vi "Set Y Voltage.vi"(8 "error in (no error)":errorcluster, 10 "Set y Voltage(V)":dbl, 11 "hdl in":i32) -> (0 "error out":errorcluster, 3 "hdl":i32)   [LabVIEW 2011, in "Thorlabs_MDT69xB.lvlib"]
doc: "Set the output voltage for the Y axis."
uses:
  <instrlib>/Thorlabs_MDT69xB/Thorlabs_MDT69xB.lvlib
  <instrlib>/Thorlabs_MDT69xB/Data/MDT_COMMAND_LIB_win32.dll
  <instrlib>/Thorlabs_MDT69xB/Data/MDT_COMMAND_LIB_x64.dll
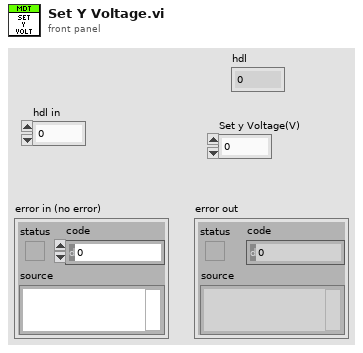
[diagram p1: front panel]
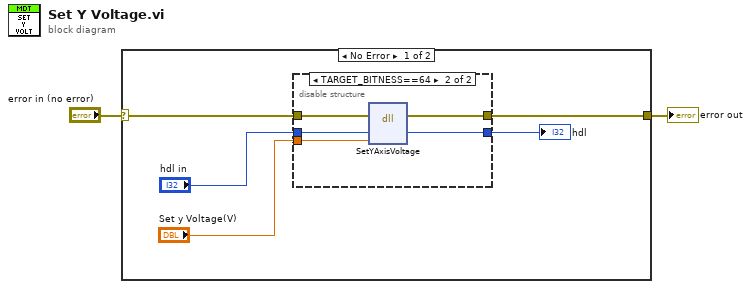
[diagram p0: block diagram]
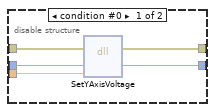
[diagram p2: hidden frame]
diagram:
  n1 = case shown="No Error" "error in (no error)" {
    selector: "error in (no error)" -> [w7 w18]
    tunnel: [w3 w18] -> w1
    frame No Error {
      n2 = disable-structure shown="TARGET_BITNESS==64" {
        disable-tunnel: w7 -> [w12 w17]
        disable-tunnel: "Set y Voltage(V)" -> [w11 w16]
        disable-tunnel: "hdl in" -> [w10 w15]
        disable-tunnel: [w9 w14] -> w4
        disable-tunnel: [w8 w13] -> w3
        frame condition #0 {
          n3 = dll-call lib="E:/Program Files (x86)/National Instruments/LabVIEW 2011/instr.lib/Thorlabs_MDT69xB/Data/MDT_COMMAND_LIB_win32.dll" fn="SetYAxisVoltage"(error in=w12, "hdl"=w10, "voltage"=w11) -> (error out=w8:errorcluster, "hdl"=w9:i32)  [unwired: 4 in, 1 out]
        }
        frame condition #1 (active) {
          n4 = dll-call lib="C:/Program Files/National Instruments/LabVIEW 2011/instr.lib/Thorlabs_MDT69xB/Data/MDT_COMMAND_LIB_x64.dll" fn="SetYAxisVoltage"(error in=w17, "hdl"=w15, "voltage"=w16) -> (error out=w13:errorcluster, "hdl"=w14:i32)  [unwired: 4 in, 1 out]
        }
      }
      "hdl" <- w4
    }
    frame Error {
    }
  }
  "error out" <- w1
